vi "CopyTreeData.vi"() -> ()   [LabVIEW 2013]
panel:
  in  "ColumnNr":i32=4
  in  "Tree 2":string[](tree)
  in  "Tree":string[](tree)
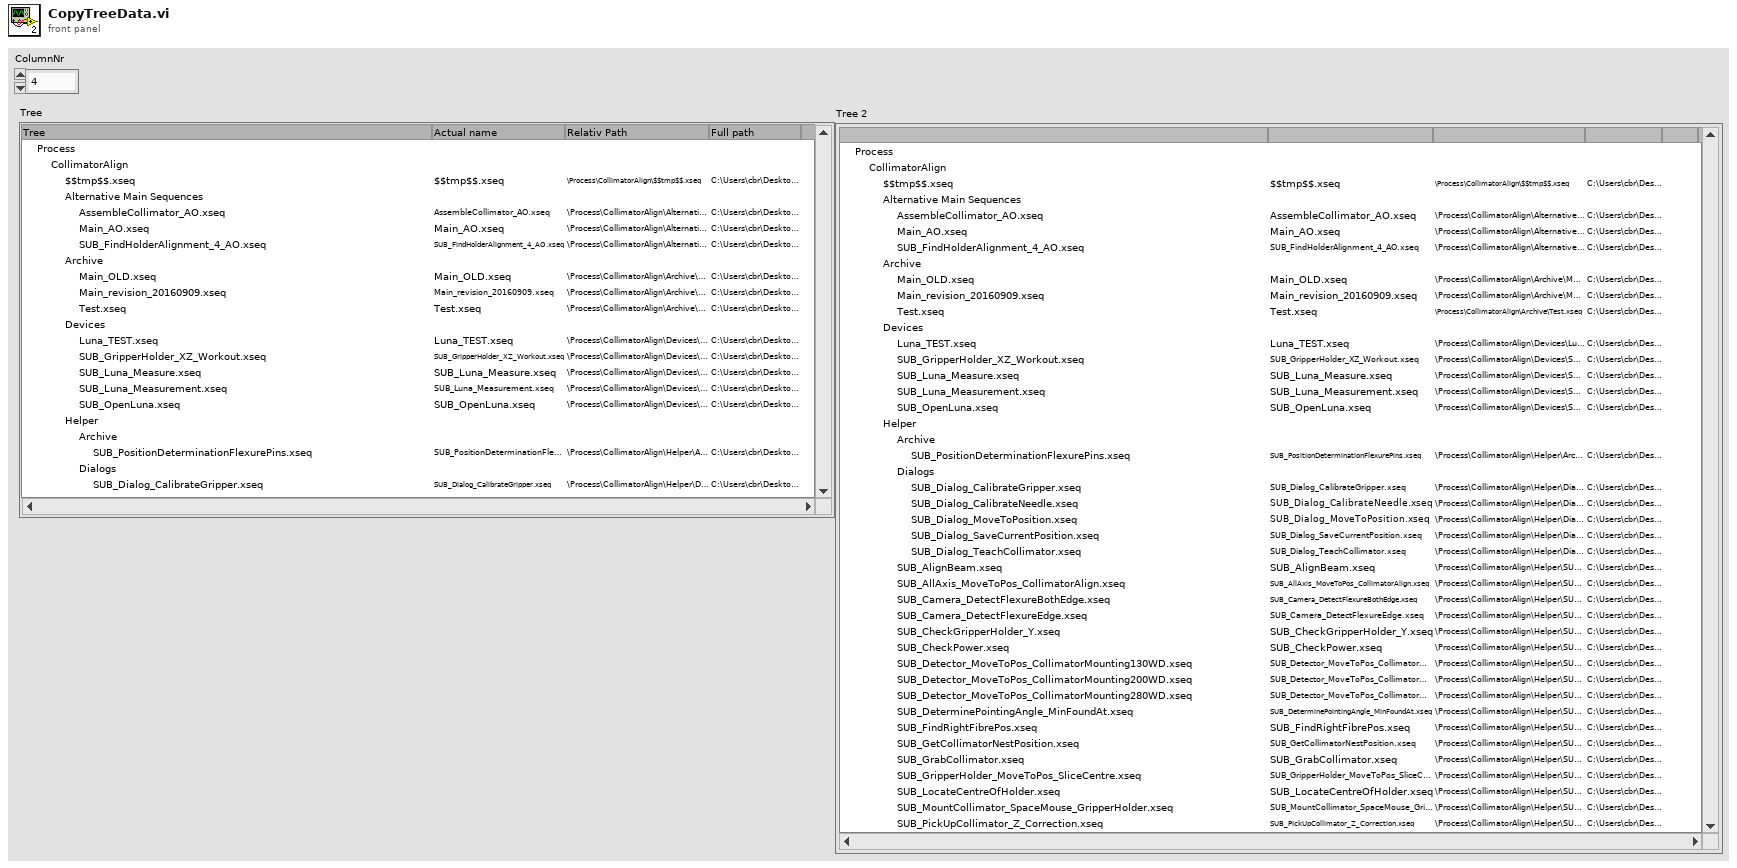
[diagram p1: front panel]
types:
  T1 = cluster{"Left Cell String":string, "Child Text":string[], "Child Tag":string, "Item Indent":i32, "Child Only?":bool, "Glyph Index":i32}
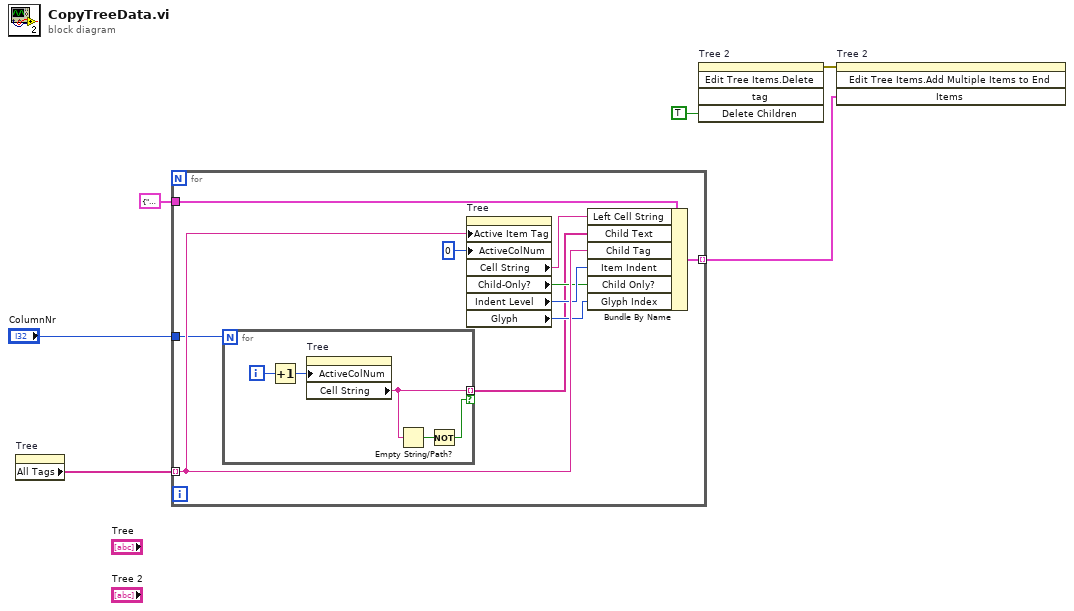
[diagram p0: block diagram]
diagram:
  n1 = property on="Tree" class="Tree (strict)"() -> ("All Tags"=w5:string[])  [unwired: 2 in, 2 out]
  n2 = for {
    tunnel: T1 {"Left Cell String"="", "Child Text"=[], "Child Tag"="", "Item Indent"=0, "Child Only?"=FALSE, "Glyph Index"=0} ("Item") -> [w16]
    tunnel: w5 -> [w15] mode=indexing
    tunnel: [w10] -> w4 mode=indexing
    tunnel: "ColumnNr" -> [w7]
    n3 = for {
      N: w7 -> [_]
      tunnel: [w19] -> w11 mode=indexing if=w17
      i -> [w21]
      n4 = Increment(x=w21) -> (x+1=w20:i32)
      n5 = property on="Tree" class="Tree (strict)"("ActiveColNum"=w20) -> ("Cell String"=w19:string)  [unwired: 2 in, 2 out]
      n6 = Empty String/Path?(string/path=w19) -> (empty?=w18:bool)
      n7 = Not(x=w18) -> (.not. x?=w17:bool)
    }
    n8 = property on="Tree" class="Tree (strict)"("Active Item Tag"=w15, "ActiveColNum"=0 ("Active Cell:Active Column Number")) -> ("Cell String"=w9:string, "Child-Only?"=w13:bool, "Indent Level"=w14:i32, "Glyph"=w12:i32)  [unwired: 2 in, 2 out]
    n9 = Bundle By Name(cluster=w16, "Left Cell String"=w9, "Child Text"=w11, "Child Tag"=w15, "Item Indent"=w14, "Child Only?"=w13, "Glyph Index"=w12) -> (w10:T1)
  }
  n10 = invoke on="Tree 2" class="Tree (strict)" method="Edit Tree Items.Delete"("Delete Children"=TRUE ("Delete Children?")) -> (error out=w2:errorcluster)  [unwired: 4 in, 4 out]
  n11 = invoke on="Tree 2" class="Tree (strict)" method="Edit Tree Items.Add Multiple Items to End"(error in=w2, "Items"=w4) -> ()  [unwired: 2 in, 4 out]
